vi "To String.vi"(8 "error in (no error)":errorcluster, 11 "Double Float in":refnum<class "Abs_I32 Integer 1D.lvclass">) -> (0 "error out":errorcluster, 2 "String":string, 3 "Double Float out":refnum<class "Abs_I32 Integer 1D.lvclass">)   [LabVIEW 2021, in "Abs_I32 Integer 1D.lvclass"]
uses:
  Abs_I32 Integer 1D.lvclass
  C:/TSA/LV_Abstract/Source/Abs_Types/Numeric 1D/Abs_Numeric_1D.lvclass
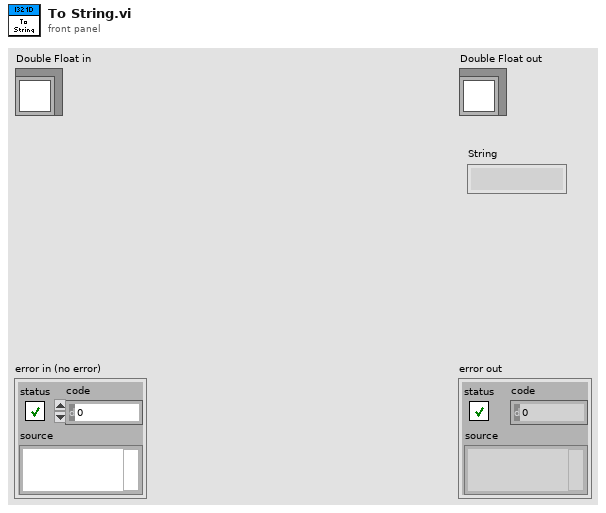
[diagram p1: front panel]
types:
  T1 = typedef "Abs_I32 Integer 1D.lvclass/Type.ctl" = i32[]
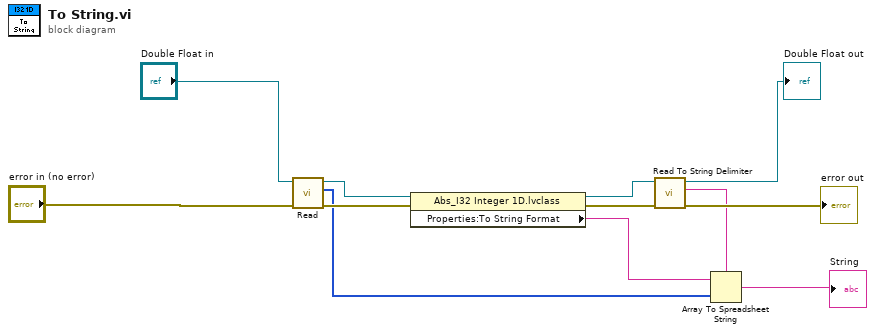
[diagram p0: block diagram]
diagram:
  n1 = call-dynamic "Read.vi"("error in (no error)"="error in (no error)", "Double Float.lvclass_340760 in"="Double Float in") -> ("error out"=w9:errorcluster, "Value"=w8:T1, "Double Float.lvclass_340760 out"=w10:refnum<class "Abs_I32 Integer 1D.lvclass">)  [unwired: 7 in]
  n2 = property class="Abs_I32 Integer 1D.lvclass"(reference=w10, error in=w9) -> (reference out=w4:refnum<class "Abs_I32 Integer 1D.lvclass">, error out=w5:errorcluster, "Properties:To String Format"=w7:string)
  n3 = call-dynamic "Read To String Delimiter.vi"("error in (no error)"=w5, "Abs_Array in"=w4) -> ("error out"=→"error out":errorcluster, "To String Delimiter"=w1:string, "Abs_Array out"=→"Double Float out":refnum<class "Abs_I32 Integer 1D.lvclass">)  [unwired: 7 in]
  n4 = Array To Spreadsheet String(delimiter (Tab)=w1, array=w8, 3:w7) -> (spreadsheet string=→"String":string)
